vi "Init.vi"(8 "error in (no error)":errorcluster caption="entrée d'erreur (pas d'erreur)", 11 "Class Multimeter Rigol DM3058 en entrée":refnum<class "Class Multimeter Rigol DM3058.lvclass">) -> (0 "error out":errorcluster caption="sortie d'erreur", 3 "Class Multimeter Rigol DM3058 en sortie":refnum<class "Class Multimeter Rigol DM3058.lvclass">)   [LabVIEW 2020, in "Library Instrument & Equipement.lvlib" / "Library Multimeter.lvlib" / "Class Multimeter Rigol DM3058.lvclass"]
uses:
  Class Multimeter Rigol DM3058.lvclass
  C:/Users/ngarcin/OneDrive - Altyor/Standard TB/Class/Multimeter/Multimeter (Default)/Class Multimeter (Default).lvclass
  Class Multimeter Rigol DM3058.lvclass/Class Multimeter Rigol DM3058.ctl
  RIGOL DM3058/RIGOL DM3058.lvlib
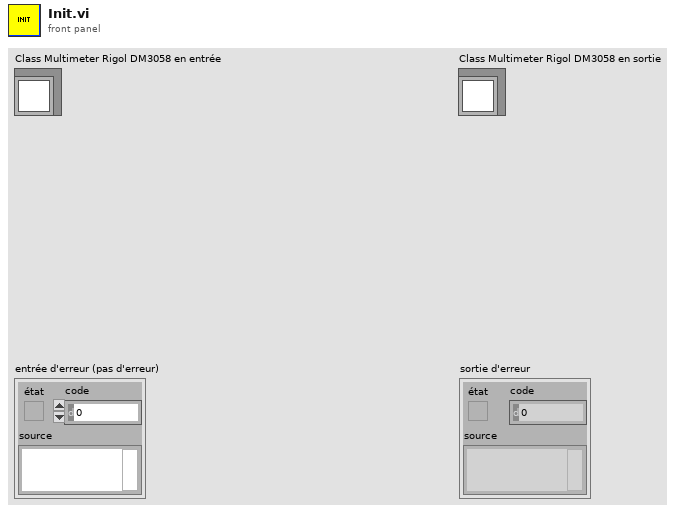
[diagram p1: front panel]
types:
  T1 = typedef "Library Commun.lvlib/Typedef Function.ctl" = enum16{"Voltmeter", "Ammeter", "Continuity", "Ohmmeter", "Frequencymeter"}
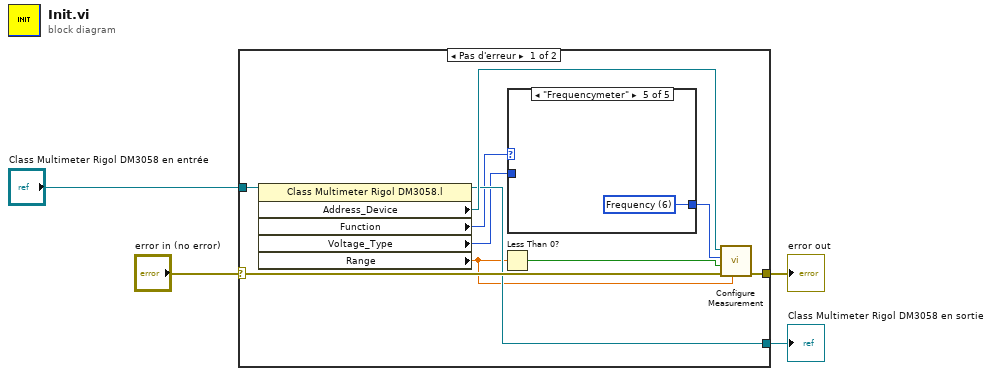
[diagram p0: block diagram]
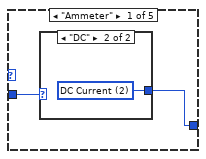
[diagram p2: hidden frame]
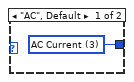
[diagram p3: hidden frame]
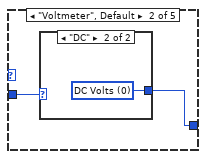
[diagram p4: hidden frame]
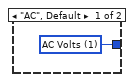
[diagram p5: hidden frame]
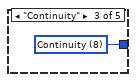
[diagram p6: hidden frame]
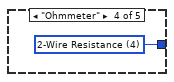
[diagram p7: hidden frame]
diagram:
  n1 = case shown="Pas d'erreur" "error in (no error)" {
    selector: "error in (no error)" -> [w13 w27]
    tunnel: [w12 w27] -> w1
    tunnel: [w10 w26] -> w3
    tunnel: "Class Multimeter Rigol DM3058 en entrée" -> [w11 w26]
    frame No Error {
      n2 = property class="Class Multimeter Rigol DM3058.l"(reference=w11) -> (reference out=w10:refnum<class "Class Multimeter Rigol DM3058.lvclass">, "Address_Device"=w14:refnum<visa-resource-name>, "Function"=w8:T1, "Voltage_Type"=w7:enum16{"AC", "DC"}, "Range"=w6:dbl)  [unwired: 1 in, 1 out]
      n3 = Less Than 0?(x=w6) -> (x < 0?=w5:bool)
      n4 = case shown="\"Frequencymeter\"" w8 {
        tunnel: [w16 w20 w23 w24 w25] -> w9
        tunnel: w7 -> [w15 w19 _ _ _]
        frame "Ammeter" {
          n5 = case shown="\"DC\"" w15 {
            tunnel: [w17 w18] -> w16
            frame "AC", Default {
              w17 = u16 3 items=["DC Volts", "AC Volts", "DC Current", "AC Current", "2-Wire Resistance", "4-Wire Resistance", "Frequency", "Period", "Continuity", "Diode", "Capacitance", "Ratio"] ("Function (0: DC Volts)")
            }
            frame "DC" {
              w18 = u16 2 items=["DC Volts", "AC Volts", "DC Current", "AC Current", "2-Wire Resistance", "4-Wire Resistance", "Frequency", "Period", "Continuity", "Diode", "Capacitance", "Ratio"] ("Function (0: DC Volts)")
            }
          }
        }
        frame "Voltmeter", Default {
          n6 = case shown="\"DC\"" w19 {
            tunnel: [w21 w22] -> w20
            frame "AC", Default {
              w21 = u16 1 items=["DC Volts", "AC Volts", "DC Current", "AC Current", "2-Wire Resistance", "4-Wire Resistance", "Frequency", "Period", "Continuity", "Diode", "Capacitance", "Ratio"] ("Function (0: DC Volts)")
            }
            frame "DC" {
              w22 = u16 0 items=["DC Volts", "AC Volts", "DC Current", "AC Current", "2-Wire Resistance", "4-Wire Resistance", "Frequency", "Period", "Continuity", "Diode", "Capacitance", "Ratio"] ("Function (0: DC Volts)")
            }
          }
        }
        frame "Continuity" {
          w23 = u16 8 items=["DC Volts", "AC Volts", "DC Current", "AC Current", "2-Wire Resistance", "4-Wire Resistance", "Frequency", "Period", "Continuity", "Diode", "Capacitance", "Ratio"] ("Function (0: DC Volts)")
        }
        frame "Ohmmeter" {
          w24 = u16 4 items=["DC Volts", "AC Volts", "DC Current", "AC Current", "2-Wire Resistance", "4-Wire Resistance", "Frequency", "Period", "Continuity", "Diode", "Capacitance", "Ratio"] ("Function (0: DC Volts)")
        }
        frame "Frequencymeter" {
          w25 = u16 6 items=["DC Volts", "AC Volts", "DC Current", "AC Current", "2-Wire Resistance", "4-Wire Resistance", "Frequency", "Period", "Continuity", "Diode", "Capacitance", "Ratio"] ("Function (0: DC Volts)")
        }
      }
      n7 = call "Configure Measurement.vi"("Manual Range (1.00)"=w6, "error in (no error)"=w13, "Auto Range (T:Enable)"=w5, "Function (0: DC Volts)"=w9, "VISA resource name"=w14) -> ("error out"=w12:errorcluster)  [unwired: 5 in, 1 out]
    }
    frame Error {
    }
  }
  "error out" <- w1
  "Class Multimeter Rigol DM3058 en sortie" <- w3
